vi "Function.vi"(8 "error in (no error)":errorcluster, 9 "Function":T2, 11 "Reference in":T1={"Device"="GPIB0::4::INSTR", "Function"="", "delay"=20}) -> (0 "error out":errorcluster, 3 "Reference out":T1={"Device"="GPIB0::4::INSTR", "Function"="", "delay"=20}, 4 "question out":string)   [LabVIEW 2021, in "Rigol DM3052.lvlib"]
uses:
  Rigol DM3052.lvlib
  Functions.ctl
  Reference.ctl
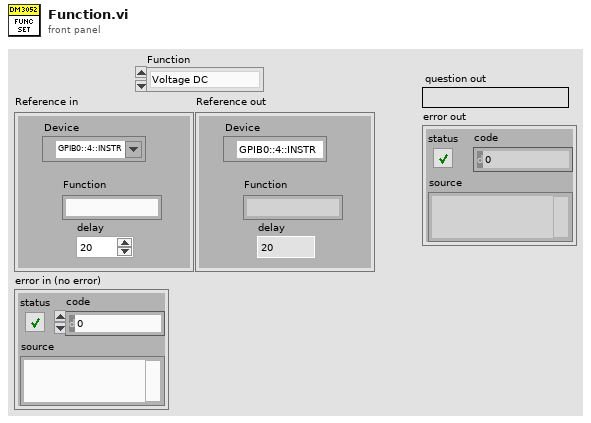
[diagram p1: front panel]
types:
  T1 = typedef "Rigol DM3052.lvlib/Reference.ctl" = cluster{"Device":refnum<visa-resource-name>, "Function":string, "delay":u32}
  T2 = typedef "Rigol DM3052.lvlib/Functions.ctl" = enum16{"Voltage DC", "Voltage AC", "Current DC", "Current AC", "Continuity", "Diode", "Resistance"}
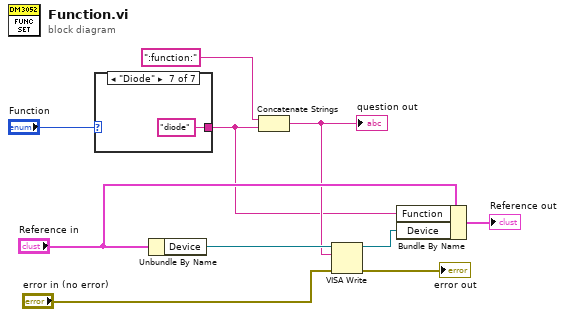
[diagram p0: block diagram]
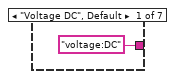
[diagram p2: hidden frame]
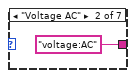
[diagram p3: hidden frame]
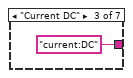
[diagram p4: hidden frame]
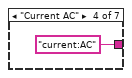
[diagram p5: hidden frame]
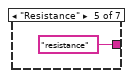
[diagram p6: hidden frame]
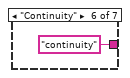
[diagram p7: hidden frame]
diagram:
  n1 = case shown="\"Diode\"" "Function" {
    tunnel: ["voltage:DC" "voltage:AC" "current:DC" "current:AC" "resistance" "continuity" "diode"] -> w1
    frame "Voltage DC", Default {
    }
    frame "Voltage AC" {
    }
    frame "Current DC" {
    }
    frame "Current AC" {
    }
    frame "Resistance" {
    }
    frame "Continuity" {
    }
    frame "Diode" {
    }
  }
  n2 = Unbundle By Name("Reference in") -> ("Device"=w8:refnum<visa-resource-name>)
  n3 = Concatenate Strings(":function:", w1) -> (w5:string)
  "question out" <- w5
  n4 = VISA Write(VISA resource name=w8, write buffer=w5, error in (no error)="error in (no error)") -> (VISA resource name out=w3:refnum<visa-resource-name>, error out=→"error out":errorcluster)  [unwired: 1 out]
  n5 = Bundle By Name(cluster="Reference in", "Function"=w1, "Device"=w3) -> (→"Reference out":T1)
